vi "rlc warning.vi"(10 "frekans index":u16, 11 "F values array":dbl[][](array[numeric])) -> ()   [LabVIEW 2014]
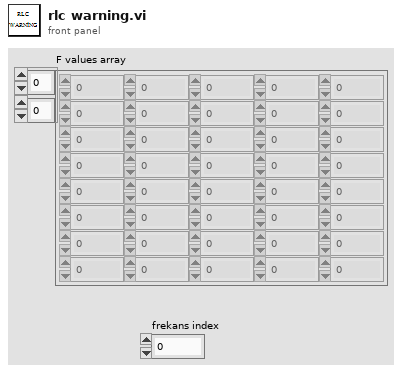
[diagram p1: front panel]
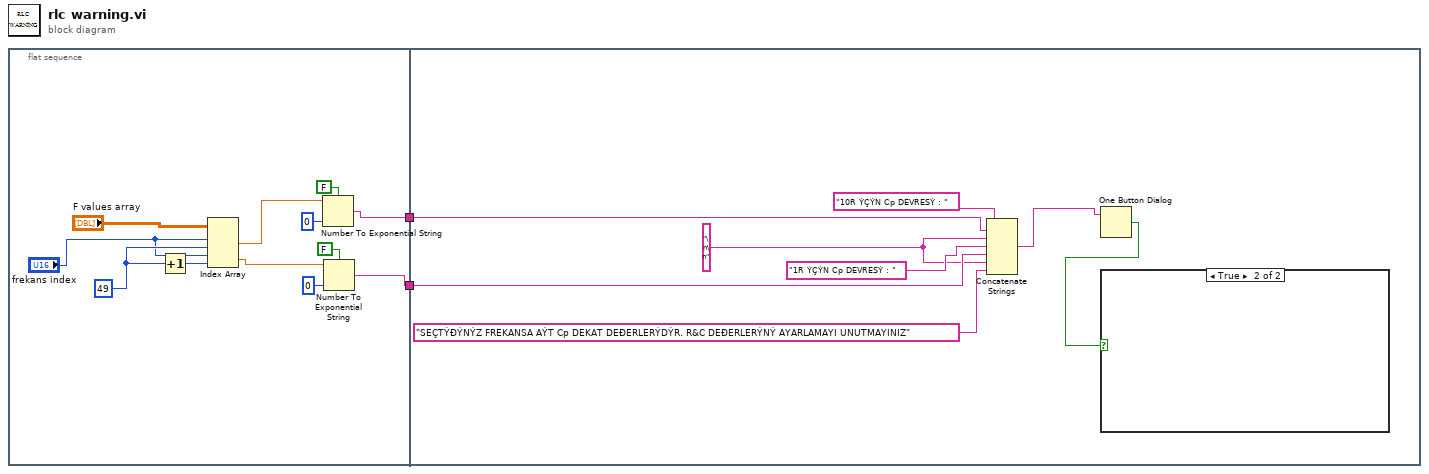
[diagram p0: block diagram]
diagram:
  n1 = flat-sequence {
    tunnel: [w4] -> w2
    tunnel: [w3] -> w1
    tunnel: w2 -> [w21]
    tunnel: w1 -> [w17]
    frame #0 {
      w13 = 49 ("disabled index (col)")
      n2 = Increment(x=w13) -> (x+1=w11:i32)
      n3 = Index Array(array="F values array", index (row) #1="frekans index", index (col) #1=w13, index (row) #2="frekans index", index (col) #2=w11) -> (element #1=w10:dbl, element #2=w7:dbl)
      n4 = Number To Exponential String(number=w10, precision (6)=i16 0, 1:FALSE ("use system decimal point (T)")) -> (E-format string=w4:string)  [unwired: 1 in]
      n5 = Number To Exponential String(number=w7, precision (6)=i16 0, 1:FALSE ("use system decimal point (T)")) -> (E-format string=w3:string)  [unwired: 1 in]
    }
    frame #1 {
      w16 = "\n\n" ("string")
      n6 = Concatenate Strings("10R ÝÇÝN Cp DEVRESÝ : " ("string"), w21, w16, "1R ÝÇÝN Cp DEVRESÝ : " ("string"), w17, w16, "SEÇTÝÐÝNÝZ FREKANSA AÝT Cp DEKAT DEÐERLERÝDÝR. R&C DEÐERLERÝNÝ AYARLAMAYI UNUTMAYINIZ" ("string")) -> (w20:string)
      n7 = One Button Dialog(message=w20) -> (true=w19:bool)  [unwired: 1 in]
      n8 = case shown="True" w19 {
        frame False {
        }
        frame True {
        }
      }
    }
  }
